vi "Encoders.vi"(6 "Motors Renum":cluster{"Num":i32, "Directly":bool, "KM":dbl}[](array[cluster]), 8 "error in (no error)":errorcluster, 9 "Reset Enc":bool, 10 "Start":bool, 11 "TitanENC in":T5) -> (0 "error out":errorcluster, 1 "RPM":T3, 2 "ENC True":T1, 3 "TitanENC out":T6, 4 "ENC/dt":T4, 5 "ENC":T1)   [LabVIEW 2020]
uses:
  <vilib>/High Genius/HG_WSI_Tookit/Dependencies/Library/TitanENC/TitanENC.lvclass
panel:
  out "ENC 2":T2
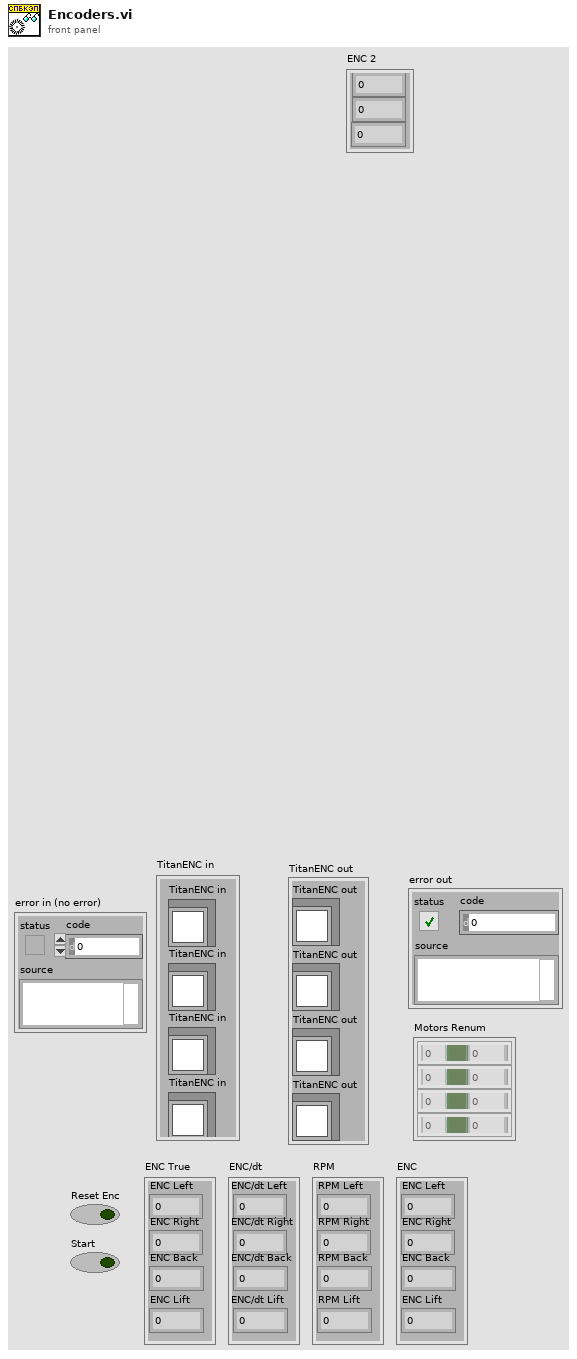
[diagram p1: front panel]
types:
  T1 = cluster{"ENC Left":i32, "ENC Right":i32, "ENC Back":i32, "ENC Lift":i32}
  T2 = cluster{"ENC Left":i32, "ENC Right":i32, "ENC Back":i32}
  T3 = cluster{"RPM Left":i32, "RPM Right":i32, "RPM Back":i32, "RPM Lift":i32}
  T4 = cluster{"ENC/dt Left":i32, "ENC/dt Right":i32, "ENC/dt Back":i32, "ENC/dt Lift":i32}
  T5 = cluster{"TitanENC in":refnum<class "TitanENC.lvclass">, "TitanENC in":refnum<class "TitanENC.lvclass">, "TitanENC in":refnum<class "TitanENC.lvclass">, "TitanENC in":refnum<class "TitanENC.lvclass">}
  T6 = cluster{"TitanENC out":refnum<class "TitanENC.lvclass">, "TitanENC out":refnum<class "TitanENC.lvclass">, "TitanENC out":refnum<class "TitanENC.lvclass">, "TitanENC out":refnum<class "TitanENC.lvclass">}
  T7 = cluster{"TitanENC 0":refnum<class "TitanENC.lvclass">, "TitanENC 1":refnum<class "TitanENC.lvclass">, "TitanENC 2":refnum<class "TitanENC.lvclass">, "TitanENC 3":refnum<class "TitanENC.lvclass">}
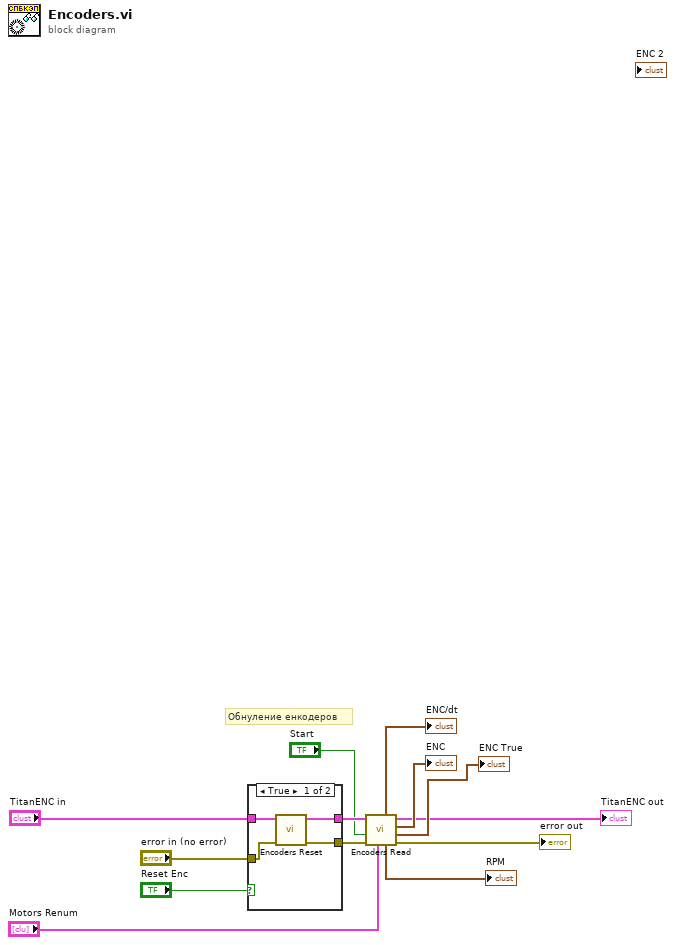
[diagram p0: block diagram]
diagram:
  # "Обнуление енкодеров"
  n1 = case shown="True" "Reset Enc" {
    tunnel: "error in (no error)" -> [w15 w18]
    tunnel: "TitanENC in" -> [w17 w19]
    tunnel: [w16 w19] -> w11
    tunnel: [w14 w18] -> w10
    frame True {
      n2 = call "Encoders Reset.vi"("error in (no error)"=w15, "TitanENC in"=w17) -> ("error out"=w14:errorcluster, "TitanENC"=w16:T7)  [unwired: 8 in]
    }
    frame False {
    }
  }
  n3 = call "Encoders Read.vi"("Motors Renum"="Motors Renum", "error in (no error)"=w10, "Start"="Start", "TitanENC in"=w11) -> ("error out"=→"error out":errorcluster, "ENC True"=→"ENC True":T1, "ENC"=→"ENC":T1, "TitanENC out"=→"TitanENC out":T6, "RPM"=→"RPM":T3, "ENC/dt"=→"ENC/dt":T4)  [unwired: 2 in]
